vi "Test Process Error Handling Outside Process Loop.vi"(8 "error in (no error)":errorcluster, 11 "Process Test In":refnum<class "Process Test.lvclass">) -> (0 "error out":errorcluster, 3 "Process Test Out":refnum<class "Process Test.lvclass">)   [LabVIEW 2020, in "Process Test.lvclass"]
uses:
  Process Test.lvclass
  Mock Error Handler/Mock Error Handler.lvclass
  Framework/Process/Process.lvclass
  <vilib>/Asteme/LUnit/Test Case.lvclass
  C:/Users/anton/Documents/GitHub/Triarc-Framework/source/Framework/Base/Base.lvclass
  C:/Users/anton/Documents/GitHub/Triarc-Framework/source/Framework Test/Mock Error Handler/Mock Error Handler.lvclass
  C:/Users/anton/Documents/GitHub/Triarc-Framework/source/Framework/Error Handler Interface/Error Handler Interface.lvclass
  C:/Users/anton/Documents/GitHub/Triarc-Framework/source/Framework Test/Base Class Test/Base Test.lvclass
  C:/Program Files (x86)/National Instruments/LabVIEW 2020/vi.lib/Asteme/LUnit/Test Case.lvclass
  C:/Users/anton/Documents/GitHub/Triarc-Framework/source/Framework Test/Process Test/Process Test.lvclass
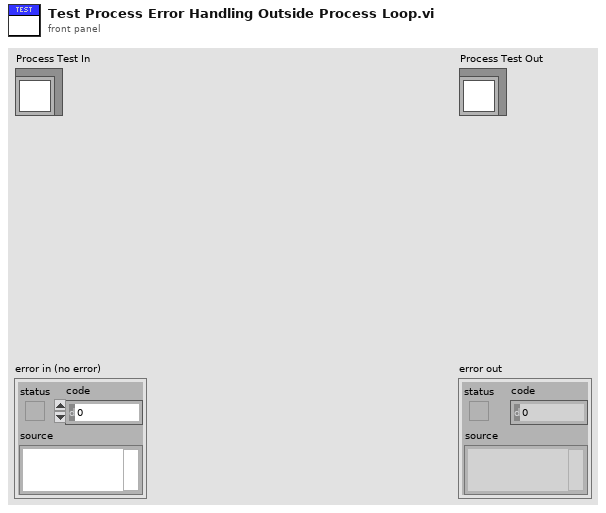
[diagram p1: front panel]
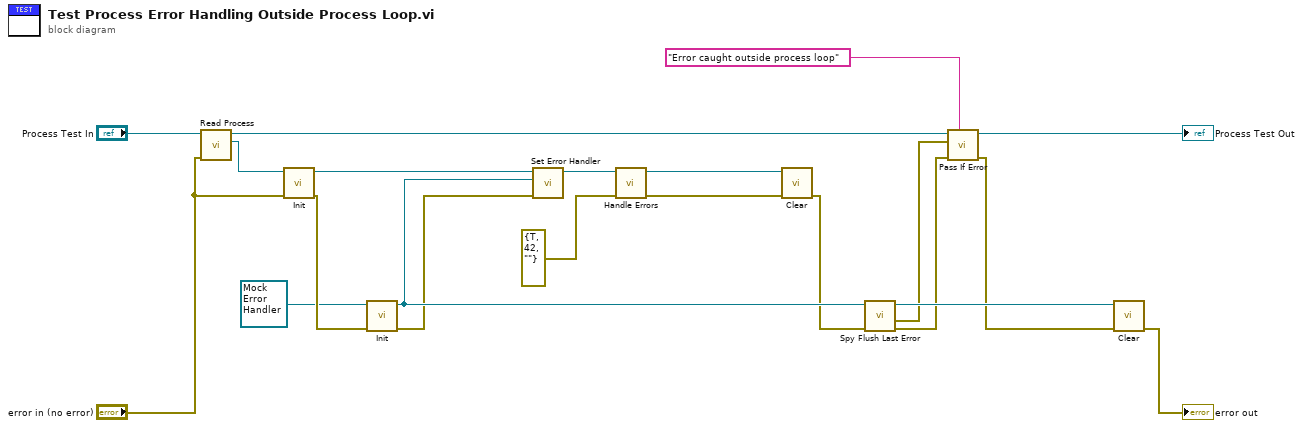
[diagram p0: block diagram]
diagram:
  n1 = call "Read Process.vi"("error in (no error)"="error in (no error)", "Process Test in"="Process Test In") -> ("Process.lvclass"=w5:refnum<class "Process.lvclass">, "Process Test out"=w4:refnum<class "Process Test.lvclass">)  [unwired: 7 in, 1 out]
  n2 = call-dynamic "Init.vi"("error in (no error)"="error in (no error)", "Process In"=w5) -> ("error out"=w20:errorcluster, "Process Out"=w18:refnum<class "Process.lvclass">)  [unwired: 8 in]
  n3 = call-dynamic "Init.vi"("error in (no error)"=w20, "Mock Error Handler In"=refnum<class "Mock Error Handler.lvclass"> refnum ("Mock Error Handler.lvclass")) -> ("error out"=w13:errorcluster, "Mock Error Handler Out"=w14:refnum<class "Mock Error Handler.lvclass">)  [unwired: 8 in]
  n4 = call "Set Error Handler.vi"("error in (no error)"=w13, "Error Handler"=w14, "Process In"=w18) -> ("Process Out"=w17:refnum<class "Process.lvclass">)  [unwired: 7 in, 1 out]
  n5 = call-dynamic "Handle Errors.vi"("error in (no error)"=errorcluster {"status"=TRUE, "code"=42, "source"=""}, "Process In"=w17) -> ("error out"=w15:errorcluster, "Process Out"=w16:refnum<class "Process.lvclass">)  [unwired: 8 in]
  n6 = call-dynamic "Clear.vi"("error in (no error)"=w15, "Process In"=w16) -> ("error out"=w10:errorcluster)  [unwired: 9 in]
  n7 = call "Spy Flush Last Error.vi"("error in (no error)"=w10, "Mock Error Handler In"=w14) -> ("error out"=w9:errorcluster, "Error"=w8:errorcluster, "Mock Error Handler Out"=w12:refnum<class "Mock Error Handler.lvclass">)  [unwired: 7 in]
  n8 = call <vilib>:"Pass If Error.vi"("Description"="Error caught outside process loop", "error in (no error)"=w9, "Assert error"=w8, "Test Case In"=w4) -> ("error out"=w7:errorcluster, "Test Case Out"=→"Process Test Out":refnum<class "Process Test.lvclass">)  [unwired: 6 in]
  n9 = call-dynamic "Clear.vi"("error in (no error)"=w7, "Mock Process In"=w12) -> ("error out"=→"error out":errorcluster)  [unwired: 9 in]
